vi "Main.vi"   [LabVIEW 2019]
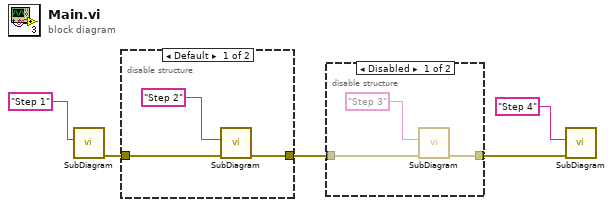
[diagram p0: block diagram]
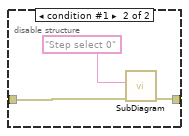
[diagram p2: hidden frame]
diagram:
  n1 = call "SubDiagram.vi"("message"="Step 1") -> ("error out"=w5:errorcluster)  [unwired: 10 in]
  n2 = disable-structure shown="Default" {
    disable-tunnel: w5 -> [w8 w10]
    disable-tunnel: [w7 w9] -> w4
    frame condition #0 (active) {
      n3 = call "SubDiagram.vi"("error in (no error)"=w8, "message"="Step 2") -> ("error out"=w7:errorcluster)  [unwired: 9 in]
    }
    frame condition #1 {
      n4 = call "SubDiagram.vi"("error in (no error)"=w10, "message"="Step select 0") -> ("error out"=w9:errorcluster)  [unwired: 9 in]
    }
  }
  n5 = disable-structure shown="Disabled" {
    disable-tunnel: w4 -> [w14 w15]
    disable-tunnel: [w13 w15] -> w3
    frame Disabled {
      n6 = call "SubDiagram.vi"("error in (no error)"=w14, "message"="Step 3") -> ("error out"=w13:errorcluster)  [unwired: 9 in]
    }
    frame Enabled {
    }
  }
  n7 = call "SubDiagram.vi"("error in (no error)"=w3, "message"="Step 4") -> ()  [unwired: 9 in, 1 out]
